vi "Read HDF5.vi"(8 "error in (no error)":errorcluster, 10 "path":path, 11 "LVtoITX in":refnum<class "LVtoITX.lvclass">) -> (0 "error out":errorcluster, 1 "Wavenames":string[](array[string]), 2 "1D Cluster Array":cluster{"array type (2D Dbl)":dbl[]}[](array[cluster]), 3 "LVtoITX out":refnum<class "LVtoITX.lvclass">, 4 "Comments":string, 6 "Igor Commands":string)   [LabVIEW 2016, in "LVtoITX.lvclass"]
uses:
  LVtoITX.lvclass
  <vilib>/addons/h5labview2/file/H5Fmode.ctl
  LVtoITX.lvclass/LVtoITX.ctl
  <vilib>/addons/h5labview2/base/lib_path.vi
  <vilib>/addons/h5labview2/base/H5Equery.vi
  <vilib>/addons/h5labview2/dataset/H5Dread.llb/H5Dread.xnode
  <vilib>/addons/h5labview2/file/H5F.lvlib
  <vilib>/addons/h5labview2/group/H5G.lvlib
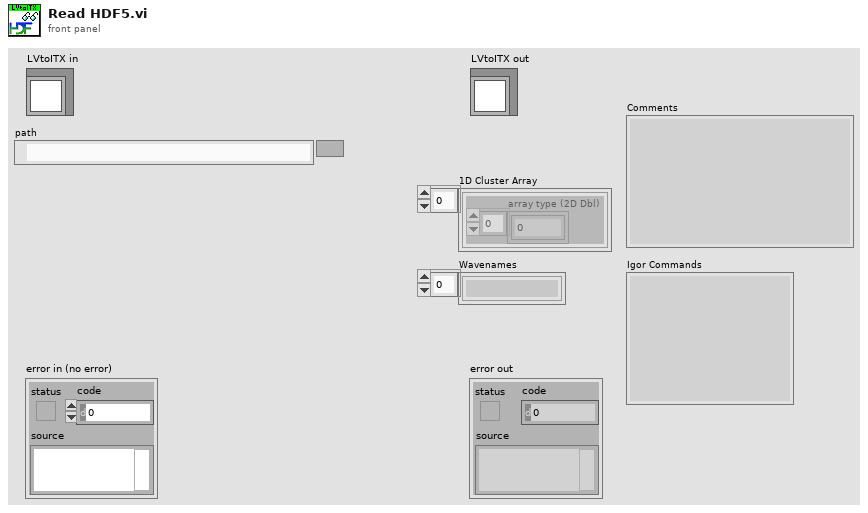
[diagram p1: front panel]
types:
  T1 = typedef "H5F.lvlib/H5Fmode.ctl" = enum16{"read-only", "read-write", "overwrite", "create new", "open or create"}
  T2 = typedef "hid_t.ctl" = i32
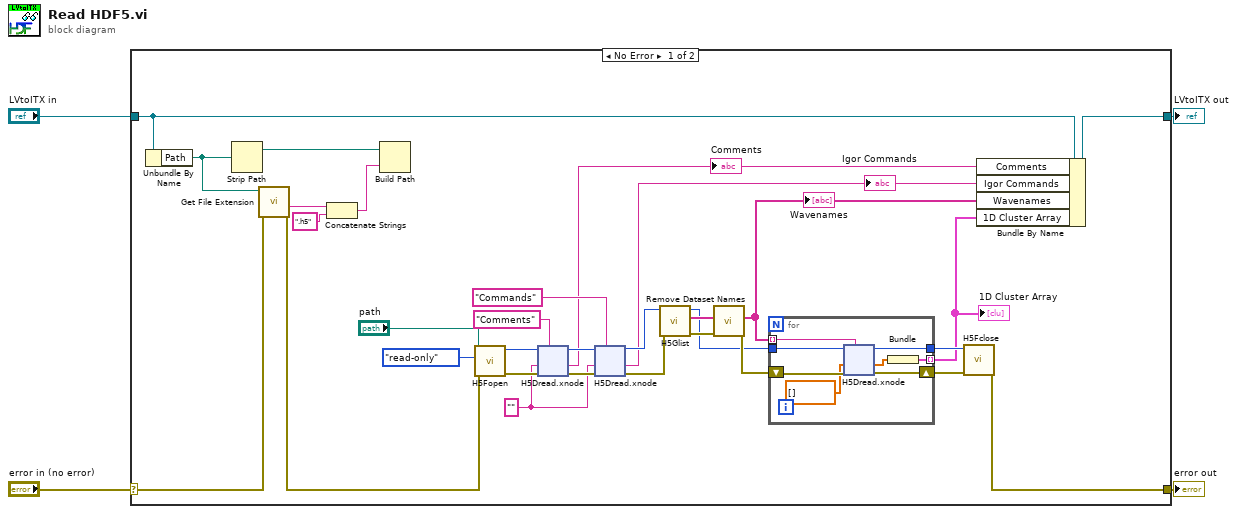
[diagram p0: block diagram]
diagram:
  n1 = case shown="No Error" "error in (no error)" {
    selector: "error in (no error)" -> [w18 w89]
    tunnel: [w24 w89] -> w1
    tunnel: [w19 w90] -> w2
    tunnel: "LVtoITX in" -> [w20 w90]
    frame No Error {
      w21 = "" ("attrib name")
      n2 = Unbundle By Name(w20) -> ("Path"=w23:path)
      n3 = Strip Path(path=w23) -> (stripped path=w32:path)  [unwired: 1 out]
      n4 = call <vilib>:"Get File Extension.vi"("error in (no error)"=w18, "file"=w23) -> ("error out"=w30:errorcluster, "filename without extension"=w34:string)  [unwired: 5 in, 3 out]
      n5 = Concatenate Strings(w34, ".h5" ("string")) -> (w31:string)
      n6 = Build Path(base path=w32, name or relative path=w31) -> ()  [unwired: 1 out]
      n7 = call <vilib>:"H5Fopen.vi"("error in (no error)"=w30, "mode (read-only)"=H5Fmode."read-only" ("mode"), "path"="path") -> ("error out"=w29:errorcluster, "ref out"=w22:T2)  [unwired: 7 in]
      n8 = xnode "H5Dread.xnode"("dataset name (this)"="Comments" ("attrib name"), "error in (no error)"=w29, "default"=w21, "ref in"=w22) -> ("error out"=w27:errorcluster, "data"=w15:string, "ref out"=w26:i32)  [unwired: 2 in, 1 out]
      "Comments" <- w15
      n9 = xnode "H5Dread.xnode"("dataset name (this)"="Commands" ("attrib name"), "error in (no error)"=w27, "default"=w21, "ref in"=w26) -> ("error out"=w7:errorcluster, "data"=w16:string, "ref out"=w17:i32)  [unwired: 2 in, 1 out]
      "Igor Commands" <- w16
      n10 = call <vilib>:"H5Glist.vi"("error in (no error)"=w7, "ref in"=w17) -> ("error out"=w10:errorcluster, "names"=w11:string[], "ref out"=w8:T2)  [unwired: 6 in, 1 out]
      n11 = call "Remove Dataset Names.vi"("error in (no error)"=w10, "Dataset Names"=w11) -> ("error out"=w9:errorcluster, "Name less Commands and Comments"=w5:string[])  [unwired: 8 in]
      "Wavenames" <- w5
      n12 = for {
        shift-right: [w43] -> w13
        shift-left: w9 -> [w42]
        tunnel: w8 -> [w41]
        tunnel: [w40] -> w12
        tunnel: w5 -> [w37] mode=indexing
        tunnel: [w36] -> w6 mode=indexing
        n13 = xnode "H5Dread.xnode"("dataset name (this)"=w37, "error in (no error)"=w42, "default"=dbl[] [] ("array type (2D Dbl)"), "ref in"=w41) -> ("error out"=w43:errorcluster, "data"=w38:dbl[], "ref out"=w40:i32)  [unwired: 2 in, 1 out]
        n14 = Bundle("data"=w38) -> (w36:cluster{"data":dbl[]})  [unwired: 1 in]
      }
      "1D Cluster Array" <- w6
      n15 = call <vilib>:"H5Fclose.vi"("error in (no error)"=w13, "ref"=w12) -> ("error out"=w24:errorcluster)  [unwired: 9 in]
      n16 = Bundle By Name(cluster=w20, "Comments"=w15, "Igor Commands"=w16, "Wavenames"=w5, "1D Cluster Array"=w6) -> (w19:refnum<class "LVtoITX.lvclass">)
    }
    frame Error {
    }
  }
  "error out" <- w1
  "LVtoITX out" <- w2
